vi "Holodrive.vi"(0 "Translation X":dbl, 5 "Translation Y":dbl, 7 "Angular":dbl, 9 "Robot Length":dbl=22.0, 11 "Robot Width":dbl=20.5) -> (2 "FL Rot":dbl, 3 "FR Rot":dbl, 4 "BL Rot":dbl, 6 "BR Rot":dbl, 10 "BR Drive":dbl, 13 "FL Drive":dbl, 14 "FR Drive":dbl, 15 "BL Drive":dbl)   [LabVIEW 2014]
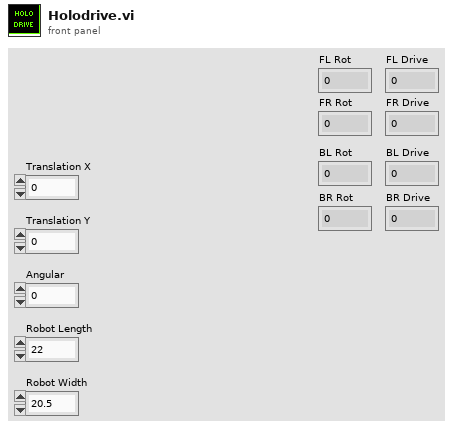
[diagram p1: front panel]
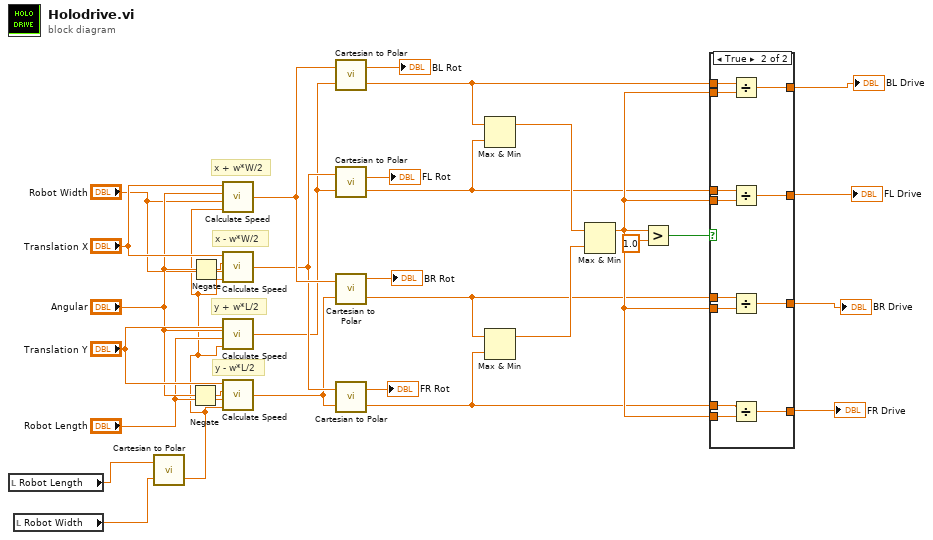
[diagram p0: block diagram]
diagram:
  # "y - w*L/2"
  # "y + w*L/2"
  # "x - w*W/2"
  # "x + w*W/2"
  n1 = local read "Robot Length"() -> (w3:dbl)
  n2 = local read "Robot Width"() -> (w2:dbl)
  n3 = call "Cartesian to Polar.vi"("y"=w2, "x"=w3) -> ("magnitude"=w1:dbl)  [unwired: 1 out]
  n4 = Negate(x="Angular") -> (-x=w29:dbl)
  n5 = Negate(x="Angular") -> (-x=w28:dbl)
  n6 = call "Calculate Speed.vi"("radius"=w1, "dimension"="Robot Width", "rotational"="Angular", "translational"="Translation X") -> ("speed"=w19:dbl)
  n7 = call "Calculate Speed.vi"("radius"=w1, "dimension"="Robot Width", "rotational"=w28, "translational"="Translation X") -> ("speed"=w18:dbl)
  n8 = call "Calculate Speed.vi"("radius"=w1, "dimension"="Robot Length", "rotational"="Angular", "translational"="Translation Y") -> ("speed"=w17:dbl)
  n9 = call "Calculate Speed.vi"("radius"=w1, "dimension"="Robot Length", "rotational"=w29, "translational"="Translation Y") -> ("speed"=w16:dbl)
  n10 = call "Cartesian to Polar.vi"("y"=w17, "x"=w19) -> ("magnitude"=w15:dbl, "angle"=→"BL Rot":dbl)
  n11 = call "Cartesian to Polar.vi"("y"=w17, "x"=w18) -> ("magnitude"=w14:dbl, "angle"=→"FL Rot":dbl)
  n12 = call "Cartesian to Polar.vi"("y"=w16, "x"=w19) -> ("magnitude"=w13:dbl, "angle"=→"BR Rot":dbl)
  n13 = call "Cartesian to Polar.vi"("y"=w16, "x"=w18) -> ("magnitude"=w12:dbl, "angle"=→"FR Rot":dbl)
  n14 = Max & Min(x=w15, y=w14) -> (max(x,y)=w24:dbl)  [unwired: 1 out]
  n15 = Max & Min(x=w13, y=w12) -> (max(x,y)=w23:dbl)  [unwired: 1 out]
  n16 = Max & Min(x=w24, y=w23) -> (max(x,y)=w20:dbl)  [unwired: 1 out]
  n17 = Greater?(x=w20, y=1.0) -> (0:w21:bool)
  n18 = case shown="True" w21 {
    tunnel: w20 -> [_ w47]
    tunnel: w20 -> [_ w46]
    tunnel: w20 -> [_ w45]
    tunnel: w20 -> [_ w44]
    tunnel: [w35 w43] -> w7
    tunnel: [w34 w42] -> w6
    tunnel: [w33 w41] -> w5
    tunnel: [w32 w40] -> w4
    tunnel: w15 -> [w35 w39]
    tunnel: w14 -> [w34 w38]
    tunnel: w13 -> [w33 w37]
    tunnel: w12 -> [w32 w36]
    frame False {
    }
    frame True {
      n19 = Divide(x=w39, y=w44) -> (x/y=w43:dbl)
      n20 = Divide(x=w38, y=w45) -> (x/y=w42:dbl)
      n21 = Divide(x=w37, y=w46) -> (x/y=w41:dbl)
      n22 = Divide(x=w36, y=w47) -> (x/y=w40:dbl)
    }
  }
  "FL Drive" <- w6
  "FR Drive" <- w4
  "BL Drive" <- w7
  "BR Drive" <- w5
